vi "Write Application Config.vi"(8 "error in (no error)":errorcluster, 9 "Config Type In":variant, 10 "Section":string, 11 "Application in":refnum<data-value>) -> (0 "error out":errorcluster, 3 "Application out":refnum<data-value>)   [LabVIEW 2015, in "Application.lvclass"]
uses:
  Application.lvclass
  Member Access/Read Path.vi
  <vilib>/Utility/config.llb/NI_LVConfig.lvlib
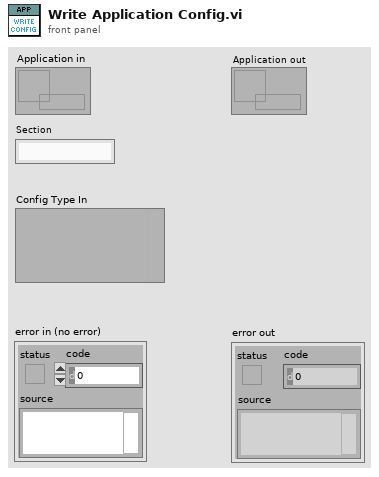
[diagram p1: front panel]
types:
  T1 = typedef "NI_LVConfig.lvlib/Config Data RefNum.ctl" = refnum<k1>
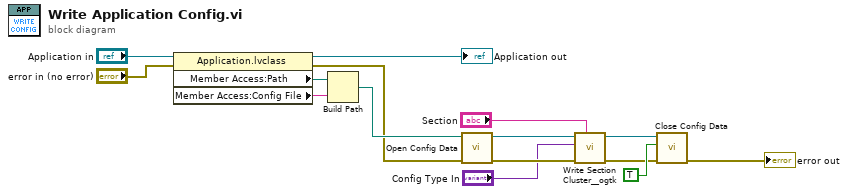
[diagram p0: block diagram]
diagram:
  n1 = property class="Application.lvclass"(reference="Application in", error in="error in (no error)") -> (reference out=→"Application out":refnum<data-value>, error out=w11:errorcluster, "Member Access:Path"=w14:path, "Member Access:Config File"=w15:string)
  n2 = Build Path(base path=w14, name or relative path=w15) -> (appended path=w13:path)
  n3 = call <vilib>:"Open Config Data.vi"("error in (no error)"=w11, "configuration file path"=w13) -> ("error out"=w7:errorcluster, "refnum"=w8:T1)  [unwired: 7 in, 1 out]
  n4 = call <userlib>:"Write Section Cluster__ogtk.vi"("section (optional)"="Section", "error in (no error)"=w7, "Section Formatted Cluster"="Config Type In", "refnum"=w8) -> ("error out"=w6:errorcluster, "dup refnum"=w5:T1)  [unwired: 6 in]
  n5 = call <vilib>:"Close Config Data.vi"("error in (no error)"=w6, "write file if changed (T)"=TRUE, "refnum"=w5) -> ("error out"=→"error out":errorcluster)  [unwired: 7 in, 1 out]
